vi "Configure Clock_5782_ver2 - Copy.vi"(8 "error in":errorcluster, 9 "User Data 1":u8, 10 "Clock Source":T1(ring), 11 "FPGA VI Reference":T2) -> (0 "error out":errorcluster, 2 "Configuration Error":bool, 3 "FPGA VI Reference out":T2)   [LabVIEW 2025]
doc: "This VI configures the clock source for the NI 5782. For execution steps, refer to the comments on the block diagram."
uses:
  Config/FPGAref_config.ctl
  <vilib>/Utility/error.llb/Error Cluster From Error Code.vi
  <vilib>/rvi/errors/niLvFpgaAdjustHostInterfaceError.vi
  <vilib>/rvi/interface/nirviReadWriteControl/nirviReadWriteControl.xnode
  <vilib>/rvi/interface/Simulation/niFpgaSimulationCallBeginRW.vi
  NiFpgaLv.dll
panel:
  # "This VI configures the clock source for the NI 5771. For execution steps, refer to the comments on the block diagram."
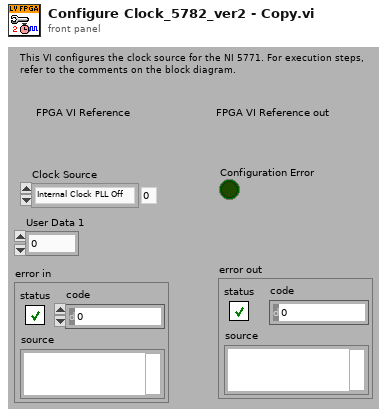
[diagram p1: front panel]
types:
  T1 = enum8{"Internal Clock PLL Off", "Internal Clock PLL On (REF IN)", "External Clock (CLK_IN)", "Internal Clock PLL On (IoModSyncClk)"}
  T2 = typedef "FPGAref_config.ctl" = refnum<k20>
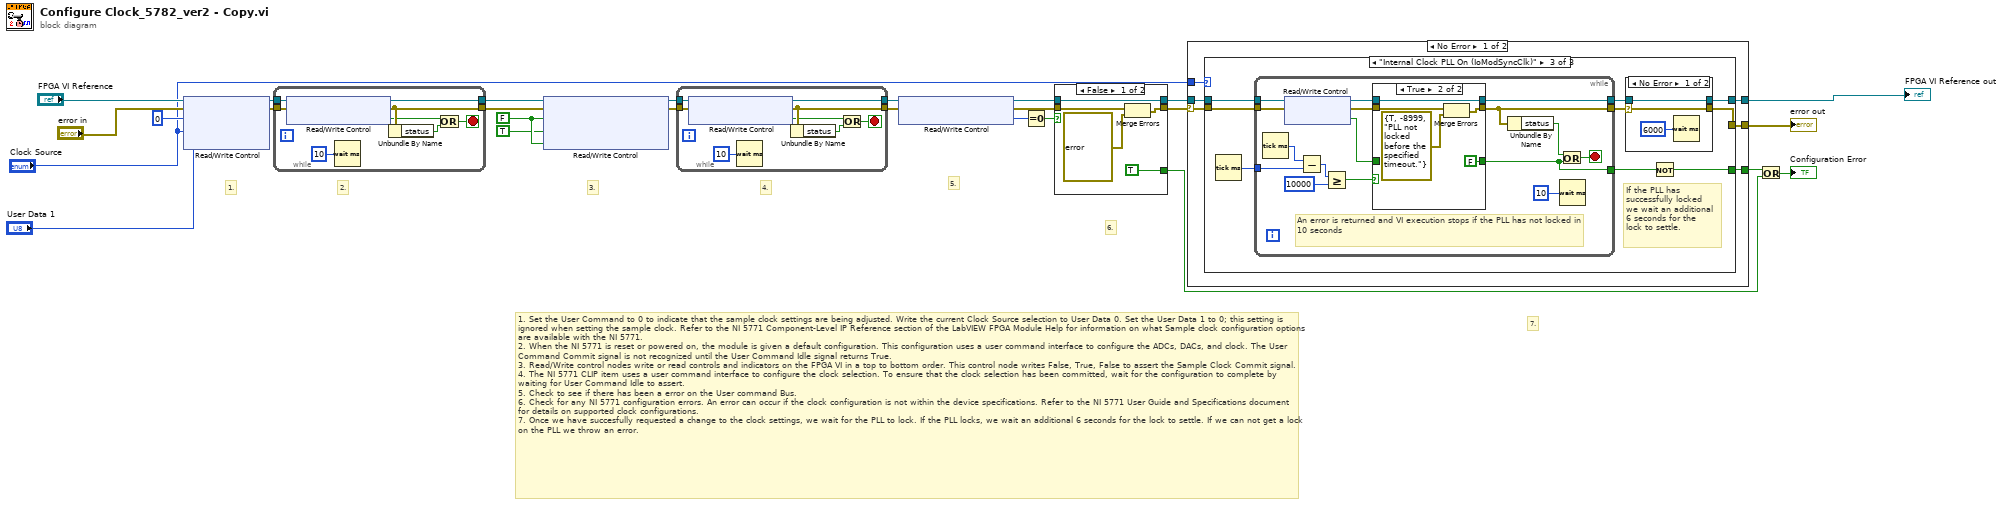
[diagram p0: block diagram]
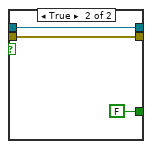
[diagram p2: hidden frame]
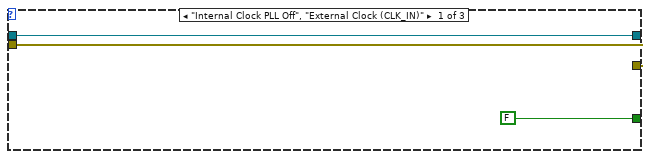
[diagram p3: hidden frame]
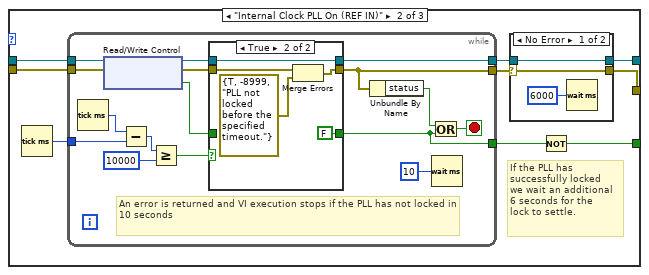
[diagram p4: hidden frame]
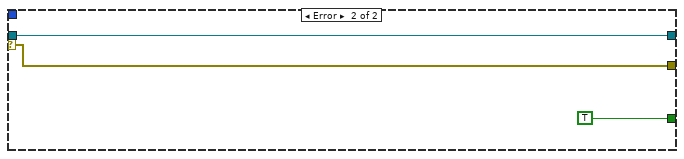
[diagram p9: hidden frame]
diagram:
  w21 = FALSE ("Sample Clock Commit")
  # "6."
  # "5."
  # "7."
  # "1. Set the User Command to 0 to indicate that the sample clock settings are being adjusted. Write the current Clock Source selection to User Data 0. Set the User Data 1 to 0; this setting is ignored when setting the sample clock. Refer to the NI 5771 Component-Level IP Reference section of the LabVIEW FPGA Module Help for information on what Sample clock configuration options are available with the NI 5771.\n2. When the NI 5771 is reset or powered on, the module is given a default configuration. This configuration uses a user command interface to configure the ADCs, DACs, and clock. The User Command Commit signal is not recognized until the User Command Idle signal returns True.\n3. Read/Write control nodes write or read controls and indicators on the FPGA VI in a top to bottom order. This control node writes False, True, False to assert the Sample Clock Commit signal.\n4. The NI 5771 CLIP item uses a user command interface to configure the clock selection. To ensure that the clock selection has been committed, wait for the configuration to complete by waiting for User Command Idle to assert.\n5. Check to see if there has been a error on the User command Bus. \n6. Check for any NI 5771 configuration errors. An error can occur if the clock configuration is not within the device specifications. Refer to the NI 5771 User Guide and Specifications document for details on supported clock configurations.\n7. Once we have succesfully requested a change to the clock settings, we wait for the PLL to lock. If the PLL locks, we wait an additional 6 seconds for the lock to settle. If we can not get a lock on the PLL we throw an error."
  # "4."
  # "3."
  # "2."
  # "1."
  n1 = xnode "Read/Write Control"("FPGA VI Reference In"="FPGA VI Reference", "error in"="error in", "User Command"=u8 0, "User Data 0"="Clock Source", "User Data 1"="User Data 1") -> ("FPGA VI Reference Out"=w25:T2, "error out"=w24:errorcluster)
  n2 = while {
    tunnel: w25 -> [w30]
    tunnel: w24 -> [w31]
    tunnel: [w28] -> w22
    tunnel: [w29] -> w23
    stop <- w32 stop-if-true
    n3 = xnode "Read/Write Control"("FPGA VI Reference In"=w30, "error in"=w31) -> ("FPGA VI Reference Out"=w29:T2, "error out"=w28:errorcluster, "User Command Idle"=w27:bool)
    n4 = Wait (ms)(milliseconds to wait=u32 10) -> ()  [unwired: 1 out]
    n5 = Unbundle By Name(w28) -> ("status"=w33:bool)
    n6 = Or(x=w27, y=w33) -> (x .or. y?=w32:bool)
  }
  n7 = xnode "Read/Write Control"("FPGA VI Reference In"=w23, "error in"=w22, "User Command Commit"=w21, "User Command Commit"=TRUE ("Sample Clock Commit"), "User Command Commit"=w21) -> ("FPGA VI Reference Out"=w19:T2, "error out"=w18:errorcluster)
  n8 = while {
    tunnel: w19 -> [w38]
    tunnel: w18 -> [w39]
    tunnel: [w36] -> w17
    tunnel: [w37] -> w16
    stop <- w40 stop-if-true
    n9 = xnode "Read/Write Control"("FPGA VI Reference In"=w38, "error in"=w39) -> ("FPGA VI Reference Out"=w37:T2, "error out"=w36:errorcluster, "User Command Idle"=w35:bool)
    n10 = Wait (ms)(milliseconds to wait=u32 10) -> ()  [unwired: 1 out]
    n11 = Unbundle By Name(w36) -> ("status"=w41:bool)
    n12 = Or(x=w35, y=w41) -> (x .or. y?=w40:bool)
  }
  n13 = xnode "Read/Write Control"("FPGA VI Reference In"=w16, "error in"=w17) -> ("FPGA VI Reference Out"=w5:T2, "error out"=w7:errorcluster, "User Command Status"=w6:u8)
  n14 = Equal To 0?(x=w6) -> (x = 0?=w4:bool)
  n15 = case shown="False" w4 {
    tunnel: [w47 w50] -> w13
    tunnel: w7 -> [w46 w50]
    tunnel: [TRUE ("Configured?") FALSE ("Configured?")] -> w8
    tunnel: w5 -> [w43 w48]
    tunnel: [w43 w48] -> w11
    frame False {
      n16 = Merge Errors(w46, errorcluster {"status"=TRUE, "code"=-8998, "source"="IO Module clock not configured correctly. Please ensure that the desired clock meets the required specifications."} ("error in")) -> (w47:errorcluster)
    }
    frame True {
    }
  }
  n17 = case shown="No Error" w13 {
    selector: w13 -> [w54 w137]
    tunnel: "Clock Source" -> [w56 _]
    tunnel: w11 -> [w55 w138]
    tunnel: [w53 w137] -> w12
    tunnel: [w52 w138] -> w1
    tunnel: [w51 TRUE ("Configured?")] -> w10
    frame No Error {
      n18 = case shown="\"Internal Clock PLL On (IoModSyncClk)\"" w56 {
        tunnel: w55 -> [w58 w67 w105]
        tunnel: w54 -> [w59 w66 w104]
        tunnel: [w59 w63 w101] -> w53
        tunnel: [w58 w64 w102] -> w52
        tunnel: [FALSE ("Configured?") w60 w98] -> w51
        frame "Internal Clock PLL Off", "External Clock (CLK_IN)" {
        }
        frame "Internal Clock PLL On (REF IN)" {
          # "If the PLL has \nsuccessfully locked \nwe wait an additional\n6 seconds for the \nlock to settle."
          n19 = Tick Count (ms)() -> (millisecond timer value=w68:u32)
          n20 = while {
            tunnel: [w87] -> w65
            tunnel: w67 -> [w84]
            tunnel: w68 -> [w80]
            tunnel: w66 -> [w78]
            tunnel: [w75] -> w62
            tunnel: [w74] -> w61
            stop <- w85 stop-if-true
            # "An error is returned and VI execution stops if the PLL has not locked in 10 seconds"
            n21 = Tick Count (ms)() -> (millisecond timer value=w81:u32)
            n22 = xnode "Read/Write Control"("FPGA VI Reference In"=w84, "error in"=w78) -> ("FPGA VI Reference Out"=w76:T2, "error out"=w82:errorcluster, "PLL Locked"=w83:bool)
            n23 = Subtract(x=w81, y=w80) -> (x-y=w79:u32)
            n24 = Greater Or Equal?(x=w79, y=u32 10000) -> (x >= y?=w88:bool)
            n25 = case shown="True" w88 {
              tunnel: [w92 FALSE ("Configured?")] -> w74
              tunnel: w83 -> [w92 _]
              tunnel: [w91 w96] -> w87
              tunnel: w82 -> [w91 w94]
              tunnel: w76 -> [w90 w93]
              tunnel: [w90 w93] -> w75
              frame False {
              }
              frame True {
                n26 = Merge Errors(w94, errorcluster {"status"=TRUE, "code"=-8999, "source"="PLL not locked before the specified timeout."} ("error in")) -> (w96:errorcluster)
              }
            }
            n27 = Unbundle By Name(w87) -> ("status"=w86:bool)
            n28 = Or(x=w86, y=w74) -> (x .or. y?=w85:bool)
            n29 = Wait (ms)(milliseconds to wait=u32 10) -> ()  [unwired: 1 out]
          }
          n30 = case shown="No Error" w65 {
            selector: w65 -> [w69 w73]
            tunnel: w62 -> [w70 w72]
            tunnel: [w70 w72] -> w64
            tunnel: [w69 w73] -> w63
            frame No Error {
              n31 = Wait (ms)(milliseconds to wait=u32 6000) -> ()  [unwired: 1 out]
            }
            frame Error {
            }
          }
          n32 = Not(x=w61) -> (.not. x?=w60:bool)
        }
        frame "Internal Clock PLL On (IoModSyncClk)" {
          # "If the PLL has \nsuccessfully locked \nwe wait an additional\n6 seconds for the \nlock to settle."
          n33 = Tick Count (ms)() -> (millisecond timer value=w106:u32)
          n34 = while {
            tunnel: [w125] -> w103
            tunnel: w105 -> [w122]
            tunnel: w106 -> [w118]
            tunnel: w104 -> [w116]
            tunnel: [w113] -> w100
            tunnel: [w112] -> w99
            stop <- w123 stop-if-true
            # "An error is returned and VI execution stops if the PLL has not locked in 10 seconds"
            n35 = Tick Count (ms)() -> (millisecond timer value=w119:u32)
            n36 = xnode "Read/Write Control"("FPGA VI Reference In"=w122, "error in"=w116) -> ("FPGA VI Reference Out"=w114:T2, "error out"=w120:errorcluster, "PLL Locked"=w121:bool)
            n37 = Subtract(x=w119, y=w118) -> (x-y=w117:u32)
            n38 = Greater Or Equal?(x=w117, y=u32 10000) -> (x >= y?=w126:bool)
            n39 = case shown="True" w126 {
              tunnel: [w130 FALSE ("Configured?")] -> w112
              tunnel: w121 -> [w130 _]
              tunnel: [w129 w134] -> w125
              tunnel: w120 -> [w129 w132]
              tunnel: w114 -> [w128 w131]
              tunnel: [w128 w131] -> w113
              frame False {
              }
              frame True {
                n40 = Merge Errors(w132, errorcluster {"status"=TRUE, "code"=-8999, "source"="PLL not locked before the specified timeout."} ("error in")) -> (w134:errorcluster)
              }
            }
            n41 = Unbundle By Name(w125) -> ("status"=w124:bool)
            n42 = Or(x=w124, y=w112) -> (x .or. y?=w123:bool)
            n43 = Wait (ms)(milliseconds to wait=u32 10) -> ()  [unwired: 1 out]
          }
          n44 = case shown="No Error" w103 {
            selector: w103 -> [w107 w111]
            tunnel: w100 -> [w108 w110]
            tunnel: [w108 w110] -> w102
            tunnel: [w107 w111] -> w101
            frame No Error {
              n45 = Wait (ms)(milliseconds to wait=u32 6000) -> ()  [unwired: 1 out]
            }
            frame Error {
            }
          }
          n46 = Not(x=w99) -> (.not. x?=w98:bool)
        }
      }
    }
    frame Error {
    }
  }
  "error out" <- w12
  "FPGA VI Reference out" <- w1
  n47 = Or(x=w10, y=w8) -> (x .or. y?=→"Configuration Error":bool)
